vi "CameraSetTimeout.vi"(8 "error in (no error)":errorcluster, 10 "Timeout":u32=1000, 11 "IMAQdx in":refnum<class "IMAQdx_Flea3_Firewire.lvclass">) -> (0 "error out":errorcluster, 2 "Timeout set":u32, 3 "IMAQdx out":refnum<class "IMAQdx_Flea3_Firewire.lvclass">)   [LabVIEW 2012, in "IMAQdx_Flea3_Firewire.lvclass"]
uses:
  <userlib>/bias2/classes/IMAQdx_Flea3_Firewire/IMAQdx_Flea3_Firewire.lvclass
  <vilib>/vision/driver/IMAQdx.llb/IMAQdx Acquisition Mode.ctl
  <userlib>/bias2/classes/IMAQdx_Flea3_Firewire/IMAQdx_Flea3_Firewire.lvclass/IMAQdx_Flea3_Firewire.ctl
  <resource>/objmgr/imaqdx.rc
  <vilib>/vision/driver/NI_Vision_Acquisition_Software.lvlib
panel:
  # "Camera Configuration"
  # "Remember, all settings and defaults can be configured in MAX"
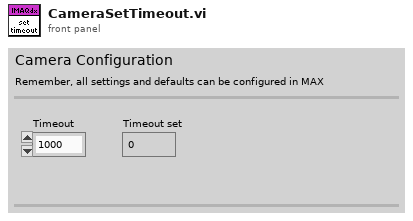
[diagram p1: front panel]
types:
  T1 = typedef "NI_Vision_Acquisition_Software.lvlib/IMAQdx Acquisition Mode.ctl" = enum32{"One Shot", "Continuous"}
  T2 = typedef "IMAQdx.ctl" = refnum<k21>
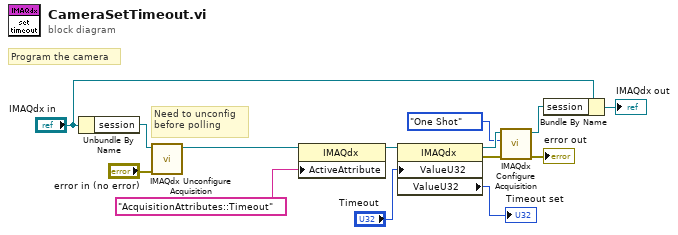
[diagram p0: block diagram]
diagram:
  # "Need to unconfig\nbefore polling"
  # "Program the camera"
  n1 = Unbundle By Name("IMAQdx in") -> ("session"=w14:refnum<k21>)
  n2 = call <vilib>:"IMAQdx Unconfigure Acquisition.vi"("error in"="error in (no error)", "Session In"=w14) -> ("Session Out"=w9:T2)  [unwired: 8 in, 1 out]
  n3 = property class="IMAQdx"(reference=w9, "ActiveAttribute"="AcquisitionAttributes::Timeout") -> (reference out=w5:T2)  [unwired: 1 in, 1 out]
  n4 = property class="IMAQdx"(reference=w5, "ValueU32"="Timeout") -> (reference out=w12:T2, error out=w2:errorcluster, "ValueU32"=→"Timeout set":u32)  [unwired: 1 in]
  n5 = call <vilib>:"IMAQdx Configure Acquisition.vi"("error in"=w2, "Continuous?"=IMAQdx_Acquisition_Mode."One Shot", "Session In"=w12) -> ("error out"=→"error out":errorcluster, "Session Out"=w8:T2)  [unwired: 7 in]
  n6 = Bundle By Name(cluster="IMAQdx in", "session"=w8) -> (→"IMAQdx out":refnum<class "IMAQdx_Flea3_Firewire.lvclass">)
